vi "Reinitialize.vi"(8 "error in (no error)":errorcluster, 11 "VI Probe in":refnum<class "PL MKS VI Probe.lvclass">) -> (0 "error out":errorcluster, 3 "VI Probe out":refnum<class "PL MKS VI Probe.lvclass">)   [LabVIEW 2015, in "PL MKS VI Probe.lvclass"]
doc: "Reinitializes connection to device based on previously specified settings."
uses:
  PL MKS VI Probe.lvclass
  PL MKS VI Probe.lvclass/PL MKS VI Probe.ctl
  <vilib>/Instr/_visa.llb/VISA Configure Serial Port (Instr).vi
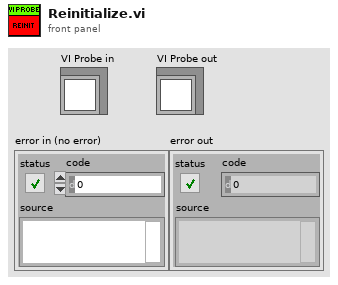
[diagram p1: front panel]
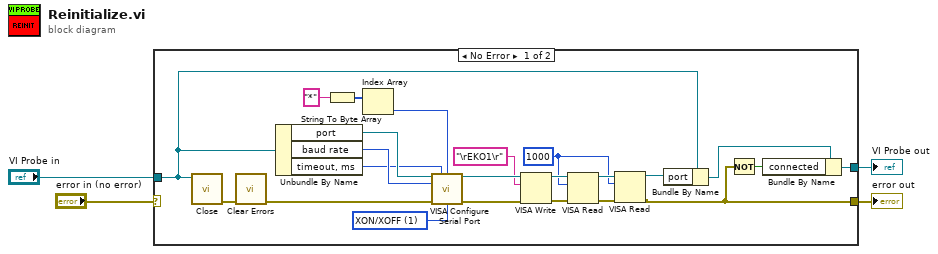
[diagram p0: block diagram]
diagram:
  n1 = case shown="No Error" "error in (no error)" {
    selector: "error in (no error)" -> [_ w28]
    tunnel: "VI Probe in" -> [w27 w29]
    tunnel: [w24 w29] -> w3
    tunnel: [w5 w28] -> w2
    frame No Error {
      w7 = u32 1000 ("byte count")
      w18 = u16 1 items=["None", "XON/XOFF", "RTS/CTS", "XON/XOFF & RTS/CTS", "DTR/DSR", "XON/XOFF & DTR/DSR"] ("flow control (0:none)")
      n2 = call "Close.vi"("VI Probe in"=w27) -> ("error out"=w20:errorcluster)  [unwired: 10 in]
      n3 = call <vilib>:"Clear Errors.vi"("error in (no error)"=w20) -> ("error out"=w19:errorcluster)  [unwired: 5 in, 1 out]
      n4 = Unbundle By Name(w27) -> ("port"=w22:refnum<visa-resource-name>, "baud rate"=w23:u32, "timeout, ms"=w21:u32)
      n5 = String To Byte Array(string="*" ("write buffer")) -> (unsigned byte array=w17:u8[])
      n6 = Index Array(array=w17) -> (element=w15:u8)  [unwired: 1 in]
      n7 = call-poly "VISA Configure Serial Port"("VISA resource name"=w22, "timeout (10sec)"=w21, "termination char\n(0xA = '\\n' = LF)"=w15, "baud rate (9600)"=w23, "error in (no error)"=w19, "flow control (0:none)"=w18) -> ("VISA resource name out"=w14:refnum<visa-resource-name>, "error out"=w13:errorcluster)  [unwired: 8 in]
      n8 = VISA Write(VISA resource name=w14, write buffer="\rEKO1\r", error in (no error)=w13) -> (VISA resource name out=w11:refnum<visa-resource-name>, error out=w10:errorcluster)  [unwired: 1 out]
      n9 = VISA Read(VISA resource name=w11, byte count=w7, error in (no error)=w10) -> (VISA resource name out=w8:refnum<visa-resource-name>, error out=w9:errorcluster)  [unwired: 2 out]
      n10 = VISA Read(VISA resource name=w8, byte count=w7, error in (no error)=w9) -> (VISA resource name out=w6:refnum<visa-resource-name>, error out=w5:errorcluster)  [unwired: 2 out]
      n11 = Bundle By Name(cluster=w27, "port"=w6) -> (w26:refnum<class "PL MKS VI Probe.lvclass">)
      n12 = Not(x=w5) -> (.not. x?=w25:bool)
      n13 = Bundle By Name(cluster=w26, "connected"=w25) -> (w24:refnum<class "PL MKS VI Probe.lvclass">)
    }
    frame Error {
    }
  }
  "VI Probe out" <- w3
  "error out" <- w2
